vi "HeaderAction.vi"(0 "InstrClass":refnum<class "YokoGS200.lvclass"> caption="DNL_LabVIEW Object in", 11 "error in (no error)":errorcluster caption="entrée d'erreur (pas d'erreur)") -> (4 "InstrClassOut":refnum<class "YokoGS200.lvclass"> caption="DNL_LabVIEW Object out", 6 "DataNames":string[](array[string]), 8 "Instr Name":string, 10 "HeaderString":string, 14 "DisplayNames":string[](array[string]), 15 "error out":errorcluster caption="sortie d'erreur")   [LabVIEW 2019, in "YokoGS200.lvclass"]
uses:
  YokoGS200.lvclass
  C:/Programmes Labview/LabScanV1A/DevicesClass/BaseDevice/BaseDevice.lvclass
  YokoGS200.lvclass/YokoGS200.ctl
  BaseDevice/BaseDevice.lvclass
panel:
  in  "Ranges":T1(ring)=enum."Minimum"
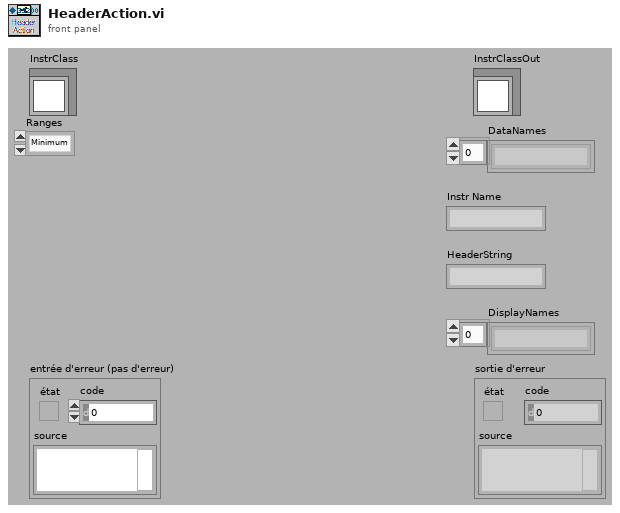
[diagram p1: front panel]
types:
  T1 = enum16{"1mA", "10mA", "100mA", "200mA", "10mV", "100mV", "1V", "10V", "30V", "Minimum", "Maximum"}
  T2 = typedef "YokoGS200.lvclass/YokoGS200_Func.ctl" = enum16{"SetVoltage (V)", "SetCurrent (A)"}
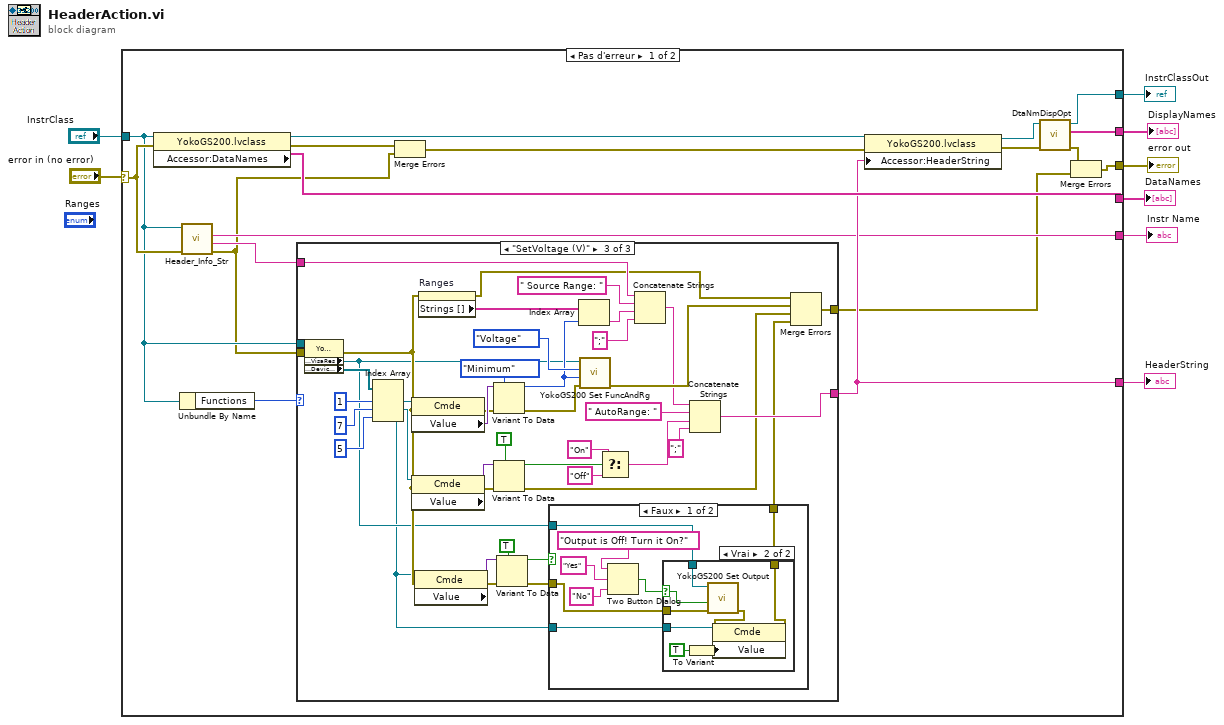
[diagram p0: block diagram]
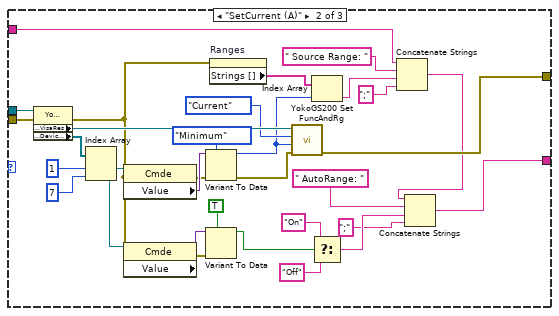
[diagram p3: hidden frame]
diagram:
  n1 = case shown="Pas d'erreur" "error in (no error)" {
    selector: "error in (no error)" -> [w14 w122]
    tunnel: [w22 _] -> w7
    tunnel: [w26 _] -> w6
    tunnel: "InstrClass" -> [w12 w123]
    tunnel: [w10 w122] -> w4
    tunnel: [w19 w123] -> w2
    tunnel: [w16 _] -> w3
    tunnel: [w17 _] -> w1
    frame No Error {
      n2 = property class="YokoGS200.lvclass"(reference=w12, error in=w14) -> (reference out=w25:refnum<class "YokoGS200.lvclass">, error out=w24:errorcluster, "Accessor:DataNames"=w26:string[])
      n3 = Unbundle By Name(w12) -> ("Functions"=w23:T2)
      n4 = call "Header_Info_Str.vi"("error in (no error)"=w14, "DefaultDev in"=w12) -> ("error out"=w11:errorcluster, "HdrInfoStr"=w15:string, "InstrumentName"=w16:string)  [unwired: 6 in, 1 out]
      n5 = case shown="\"SetVoltage (V)\"" w23 {
        tunnel: [w28 w30 w76] -> w22
        tunnel: w15 -> [w28 w44 w88]
        tunnel: w12 -> [_ w60 w103]
        tunnel: w11 -> [w27 w55 w99]
        tunnel: [w27 w43 w66] -> w9
        frame Default {
        }
        frame "SetCurrent (A)" {
          n6 = property class="YokoGS200.lvclass"(reference=w60, error in=w55) -> (error out=w40:errorcluster, "Accessor:VisaRes"=w59:refnum<visa-resource-name>, "Accessor:DeviceCtrl"=w56:refnum<vi>[])  [unwired: 1 out]
          n7 = Index Array(array=w56, index #1=1 ("index"), index #2=7 ("index")) -> (element #1=w53:refnum<vi>, element #2=w39:refnum<vi>)
          n8 = property class="Cmde"(reference=w53, error in=w40) -> (error out=w51:errorcluster, "Value"=w52:variant)  [unwired: 1 out]
          n9 = property class="Cmde"(reference=w39, error in=w40) -> (error out=w41:errorcluster, "Value"=w38:variant)  [unwired: 1 out]
          n10 = Variant To Data(error in=w51, type=T1."Minimum" ("y"), Variant=w52) -> (data=w49:T1, error out=w50:errorcluster)
          n11 = Variant To Data(error in=w41, type=TRUE, Variant=w38) -> (data=w36:bool)  [unwired: 1 out]
          n12 = property on="Ranges" class="Énum (strict)"(error in=w40) -> ("Strings []"=w47:string[])  [unwired: 1 in, 2 out]
          n13 = call <userlib>:"YokoGS200 Set FuncAndRg.vi"("error in (no error)"=w50, "Source Range"=w49, "Source Function"=enum16{"Current", "Voltage"}."Current", "VISA Rsrc"=w59) -> ("error out"=w43:errorcluster)  [unwired: 5 in, 2 out]
          n14 = Index Array(array=w47, index=w49) -> (element=w46:string)
          n15 = Select(t="On", s=w36, f="Off") -> (s? t:f=w32:string)
          n16 = Concatenate Strings(w44, " Source Range: ", w46, ";" ("string")) -> (w31:string)
          n17 = Concatenate Strings(w31, " AutoRange: ", w32, ";" ("string")) -> (w30:string)
        }
        frame "SetVoltage (V)" {
          n18 = property class="YokoGS200.lvclass"(reference=w103, error in=w99) -> (error out=w69:errorcluster, "Accessor:VisaRes"=w64:refnum<visa-resource-name>, "Accessor:DeviceCtrl"=w100:refnum<vi>[])  [unwired: 1 out]
          n19 = Index Array(array=w100, index #1=1 ("index"), index #2=7 ("index"), index #3=5 ("index")) -> (element #1=w97:refnum<vi>, element #2=w70:refnum<vi>, element #3=w61:refnum<vi>)
          n20 = property class="Cmde"(reference=w97, error in=w69) -> (error out=w95:errorcluster, "Value"=w96:variant)  [unwired: 1 out]
          n21 = property class="Cmde"(reference=w70, error in=w69) -> (error out=w85:errorcluster, "Value"=w84:variant)  [unwired: 1 out]
          n22 = property class="Cmde"(reference=w61, error in=w69) -> (error out=w71:errorcluster, "Value"=w72:variant)  [unwired: 1 out]
          n23 = property on="Ranges" class="Énum (strict)"(error in=w69) -> (error out=w65:errorcluster, "Strings []"=w91:string[])  [unwired: 1 in, 1 out]
          n24 = Variant To Data(error in=w95, type=T1."Minimum" ("y"), Variant=w96) -> (data=w93:T1, error out=w94:errorcluster)
          n25 = Variant To Data(error in=w85, type=TRUE, Variant=w84) -> (data=w82:bool, error out=w63:errorcluster)
          n26 = Variant To Data(error in=w71, type=TRUE, Variant=w72) -> (data=w68:bool, error out=w67:errorcluster)
          n27 = case shown="Faux" w68 {
            tunnel: w67 -> [w111 w121]
            tunnel: w64 -> [w110 _]
            tunnel: [w105 w121] -> w62
            tunnel: w61 -> [w104 _]
            frame False {
              n28 = Two Button Dialog(message="Output is Off! Turn it On?", 1:"No" ("F button name (\"Cancel\")"), 2:"Yes" ("T button name (\"OK\")")) -> (T button?=w106:bool)
              n29 = case shown="Vrai" w106 {
                selector: w106 -> [_ w119]
                tunnel: w111 -> [w112 w118]
                tunnel: w110 -> [_ w120]
                tunnel: [w112 w113] -> w105
                tunnel: w104 -> [_ w117]
                frame False {
                }
                frame True {
                  n30 = To Variant(anything=TRUE) -> (Variant=w115:variant)
                  n31 = call <userlib>:"YokoGS200 Set Output.vi"("error in (no error)"=w118, "Output State"=w119, "VISA Rsrc"=w120) -> ("error out"=w114:errorcluster)  [unwired: 7 in, 1 out]
                  n32 = property class="Cmde"(reference=w117, error in=w114, "Value"=w115) -> (error out=w113:errorcluster)  [unwired: 1 out]
                }
              }
            }
            frame True {
            }
          }
          n33 = Index Array(array=w91, index=w93) -> (element=w90:string)
          n34 = call <userlib>:"YokoGS200 Set FuncAndRg.vi"("error in (no error)"=w94, "Source Range"=w93, "Source Function"=enum16{"Current", "Voltage"}."Voltage", "VISA Rsrc"=w64) -> ("error out"=w87:errorcluster)  [unwired: 5 in, 2 out]
          n35 = Select(t="On", s=w82, f="Off") -> (s? t:f=w78:string)
          n36 = Concatenate Strings(w88, " Source Range: ", w90, ";" ("string")) -> (w77:string)
          n37 = Concatenate Strings(w77, " AutoRange: ", w78, ";" ("string")) -> (w76:string)
          n38 = Merge Errors(w65, w87, w63, w62) -> (w66:errorcluster)
        }
      }
      n39 = Merge Errors(w24, w11) -> (w13:errorcluster)
      n40 = property class="YokoGS200.lvclass"(reference=w25, error in=w13, "Accessor:HeaderString"=w22) -> (reference out=w18:refnum<class "YokoGS200.lvclass">, error out=w21:errorcluster)
      n41 = call "DtaNmDispOpt.vi"("error in (no error)"=w21, "BaseDevice en entrée"=w18) -> ("error out"=w20:errorcluster, "DisplayNames"=w17:string[], "BaseDevice en sortie"=w19:refnum<class "YokoGS200.lvclass">)  [unwired: 7 in]
      n42 = Merge Errors(w20, w9) -> (w10:errorcluster)
    }
    frame Error {
    }
  }
  "error out" <- w4
  "InstrClassOut" <- w2
  "DataNames" <- w6
  "HeaderString" <- w7
  "Instr Name" <- w3
  "DisplayNames" <- w1
